vi "Save Data file header and path configuration.vi"(1 "Save":bool, 2 "File name":string="Name") -> (0 "Output Path":path)   [LabVIEW 2018]
uses:
  <vilib>/Utility/file.llb/Write To Spreadsheet File (string).vi
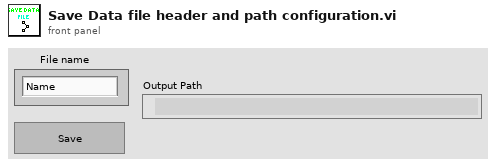
[diagram p1: front panel]
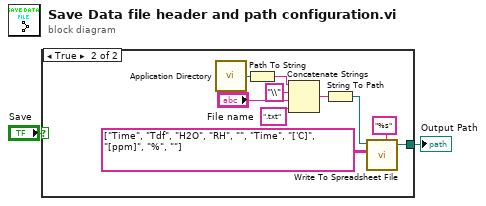
[diagram p0: block diagram]
diagram:
  n1 = case shown="True" "Save" {
    tunnel: [_ w6] -> w1
    frame False {
    }
    frame True {
      n2 = call <vilib>:"Application Directory.vi"() -> ("Application Directory"=w5:path)
      n3 = Path To String(path=w5) -> (string=w4:string)
      n4 = Concatenate Strings(w4, "\\" ("string"), "File name", ".txt" ("string")) -> (w11:string)
      n5 = String To Path(string=w11) -> (path=w12:path)
      n6 = call-poly <vilib>:"Write To Spreadsheet File.vi"("format (%s)"="%s", "2D data"=string[][] [["Time", "Tdf", "H2O", "RH", ""], ["Time", "['C]", "[ppm]", "%", ""]], "file path (dialog if empty)"=w12) -> ("new file path (Not A Path if cancelled)"=w6:path)  [unwired: 5 in]
    }
  }
  "Output Path" <- w1
